vi "lookup_node_successors.vi"(10 "node":refnum<class "Node.lvclass">, 11 "digraph":refnum<class "DiGraph.lvclass">) -> (1 "successors":refnum<class "Node.lvclass">[](array[class]), 2 "node not found?":bool)   [LabVIEW 2020, in "graph.lvlib" / "DiGraph.lvclass"]
uses:
  DiGraph.lvclass
  C:/Projects/labview-project-load-tools/source/submodules/graph-api-labview/source/api/Graph/Graph.lvclass
  Node/Node.lvclass
  Node/Node.lvclass/Node.ctl
  DiGraph.lvclass/DiGraph.ctl
  Graph/Graph.lvclass
  ca42994e-17d4-4c1a-a943-48cccf4e0eab.vi
  C:/Projects/labview-project-load-tools/source/submodules/graph-api-labview/source/api/DiGraph/DiGraph.lvclass
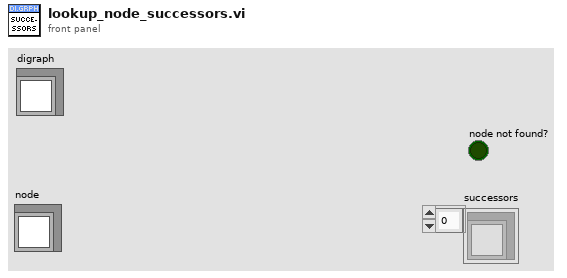
[diagram p1: front panel]
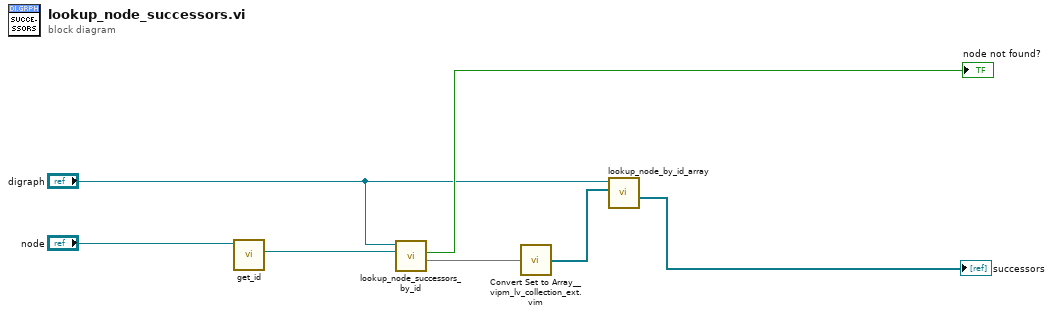
[diagram p0: block diagram]
diagram:
  n1 = call "get_id.vi"("node"="node") -> ("node-id"=w5:refnum<class "ID.lvclass">)  [unwired: 10 in]
  n2 = call "lookup_node_successors_by_id.vi"("node-id"=w5, "self"="digraph") -> ("successor_ids"=w3:set{refnum<class "ID.lvclass">}, "node not found?"=→"node not found?":bool)  [unwired: 8 in]
  n3 = call "Convert Set to Array__vipm_lv_collection_ext.vim"("set"=w3) -> ("array"=w2:refnum<class "ID.lvclass">[])  [unwired: 8 in]
  n4 = call "lookup_node_by_id_array.vi"("node_ids"=w2, "graph"="digraph") -> ("nodes"=→"successors":refnum<class "Node.lvclass">[])  [unwired: 8 in, 1 out]
